vi "checkBeginNormalDefensiveWithDuelistPlay.vi"(8 "error in (no error)":errorcluster, 10 "Game":refnum<class "Game.lvclass">, 11 "NormalDefensiveWithDuelistPlay in":refnum<class "NormalDefensiveWithDuelistPlay.lvclass">) -> (0 "error out":errorcluster, 2 "Boolean":bool, 3 "NormalDefensiveWithDuelistPlay out":refnum<class "NormalDefensiveWithDuelistPlay.lvclass">)   [LabVIEW 2018, in "NormalDefensiveWithDuelistPlay.lvclass"]
uses:
  NormalDefensiveWithDuelistPlay.lvclass
  Game_class/Game.lvclass
  Game_class/Game.lvclass/Game.ctl
  Events_class/Events.lvclass/Events.ctl
  Object_class/Object.lvclass/Object.ctl
  Ball_class/Ball.lvclass/Ball.ctl
  Game_class/Read EventsRef.vi
  Game_class/Read BallRef.vi
  Game_class/Read Parameters.lvclass.vi
  Game_class/Read FieldRef.vi
  Game_class/Read Utilities.lvclass.vi
  Object_class/Read x.vi
  Object_class/Read y.vi
  Ball_class/Read v_x.vi
  Ball_class/Read v_y.vi
  Events_class/Read ball_inside_our_goalie_area.vi
  Events_class/Read ball_out.vi
  Ball_class/Ball.lvclass
  C:/Users/anton/Desktop/roboime/CondicoesPlays/SSL_AI/Object_class/Object.lvclass
  Events_class/Events.lvclass
  Parameters_class/Parameters.lvclass
  Field_class/Field.lvclass
  Utilities_class/Utilities.lvclass
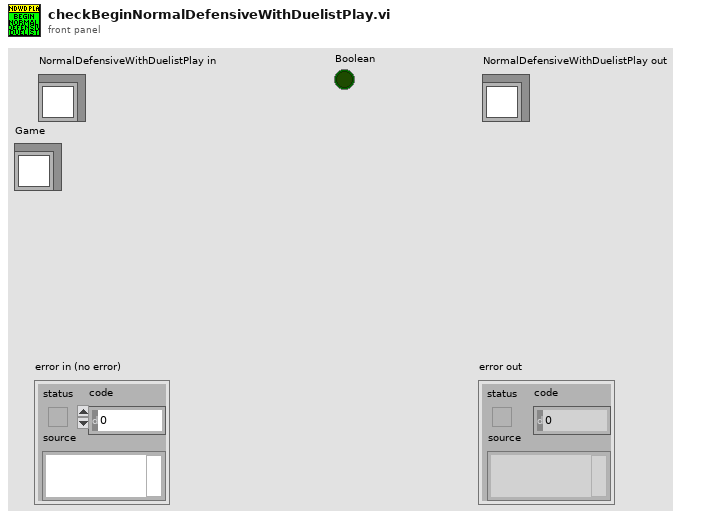
[diagram p1: front panel]
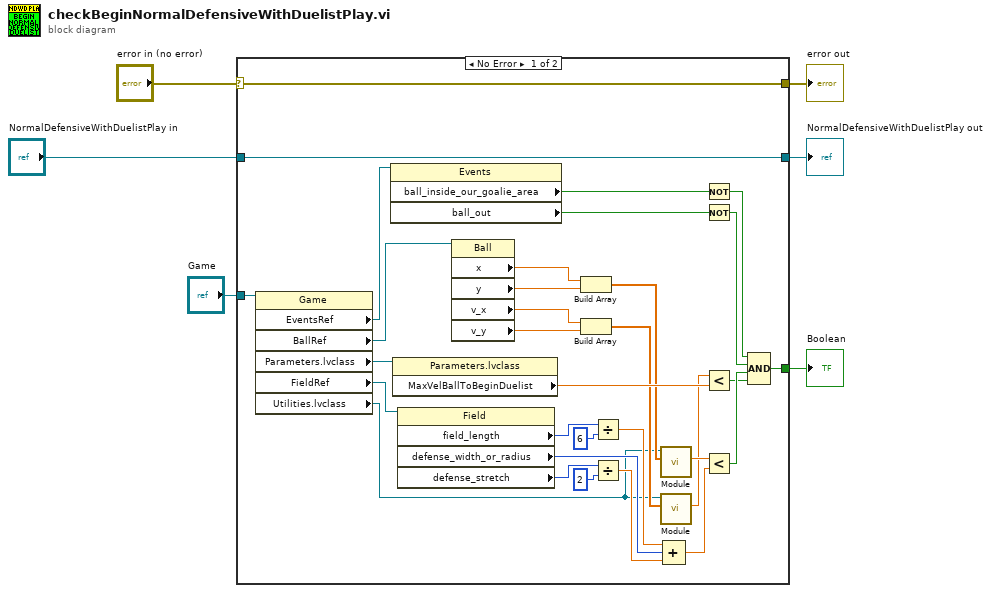
[diagram p0: block diagram]
diagram:
  n1 = case shown="No Error" "error in (no error)" {
    selector: "error in (no error)" -> [w37 w40]
    tunnel: [w37 w40] -> w5
    tunnel: [w38 w39] -> w3
    tunnel: "NormalDefensiveWithDuelistPlay in" -> [w38 w39]
    tunnel: "Game" -> [w36 _]
    tunnel: [w30 _] -> w1
    frame No Error {
      n2 = property class="Game"(reference=w36) -> ("EventsRef"=w35:refnum<class "Events.lvclass">, "BallRef"=w29:refnum<class "Ball.lvclass">, "Parameters.lvclass"=w26:refnum<class "Parameters.lvclass">, "FieldRef"=w22:refnum<class "Field.lvclass">, "Utilities.lvclass"=w7:refnum<class "Utilities.lvclass">)  [unwired: 1 in, 2 out]
      n3 = property class="Events"(reference=w35) -> ("ball_inside_our_goalie_area"=w34:bool, "ball_out"=w33:bool)  [unwired: 1 in, 2 out]
      n4 = property class="Parameters.lvclass"(reference=w26) -> ("MaxVelBallToBeginDuelist"=w23:dbl)  [unwired: 1 in, 2 out]
      n5 = property class="Field"(reference=w22) -> ("field_length"=w21:i32, "defense_width_or_radius"=w18:i32, "defense_stretch"=w16:i32)  [unwired: 1 in, 2 out]
      n6 = property class="Ball"(reference=w29) -> ("x"=w28:dbl, "y"=w27:dbl, "v_x"=w25:dbl, "v_y"=w24:dbl)  [unwired: 1 in, 2 out]
      n7 = Build Array(w28, w27) -> (w11:dbl[])
      n8 = Build Array(w25, w24) -> (w9:dbl[])
      n9 = Divide(x=w21, y=6) -> (x/y=w19:dbl)
      n10 = Divide(x=w16, y=2) -> (x/y=w15:dbl)
      n11 = call-dynamic "Module.vi"("2D vector"=w11, "Utilities in"=w7) -> ("Modulo"=w10:dbl)  [unwired: 7 in, 2 out]
      n12 = call-dynamic "Module.vi"("2D vector"=w9, "Utilities in"=w7) -> ("Modulo"=w8:dbl)  [unwired: 7 in, 2 out]
      n13 = Compound Arithmetic op=ADD(w19, w18, w15) -> (w14:dbl)
      n14 = Not(x=w34) -> (.not. x?=w32:bool)
      n15 = Not(x=w33) -> (.not. x?=w31:bool)
      n16 = Less?(x=w8, y=w23) -> (x < y?=w12:bool)
      n17 = Less?(x=w10, y=w14) -> (x < y?=w13:bool)
      n18 = Compound Arithmetic op=AND(w32, w31, w13, w12) -> (w30:bool)
    }
    frame Error {
    }
  }
  "error out" <- w5
  "NormalDefensiveWithDuelistPlay out" <- w3
  "Boolean" <- w1
